vi "State Enter.vi"(11 "State in":refnum<class "State.lvclass">) -> (0 "error out":errorcluster, 3 "State out":refnum<class "State.lvclass">)   [LabVIEW 2021, in "State.lvclass"]
uses:
  State.lvclass
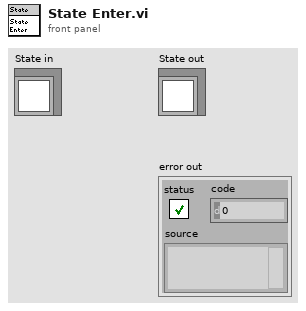
[diagram p1: front panel]
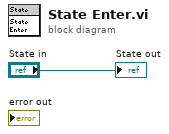
[diagram p0: block diagram]
diagram:
  "State out" <- "State in"
